vi "Untitled 1.vi"   [LabVIEW 2014]
uses:
  <vilib>/FTP/NI_FTP.lvlib
types:
  T1 = typedef "NI_FTP.lvlib/FTP Session.ctl" = refnum<k5>
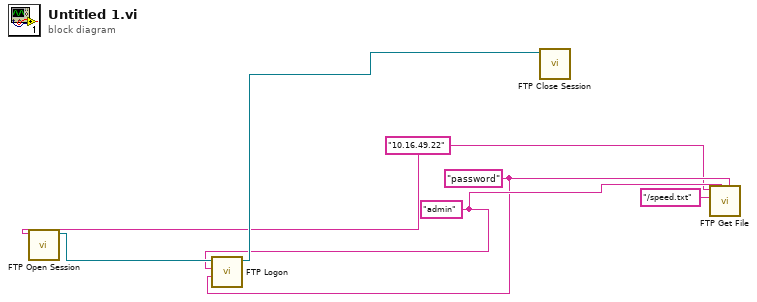
[diagram p0: block diagram]
diagram:
  w2 = "10.16.49.22" ("host")
  w3 = "password" ("password")
  w4 = "admin" ("user")
  n1 = call <vilib>:"FTP Open Session.vi"("address"=w2) -> ("ftp session"=w6:T1)  [unwired: 7 in, 3 out]
  n2 = call <vilib>:"FTP Logon.vi"("password"=w3, "user"=w4, "ftp session"=w6) -> ("ftp session out"=w5:T1)  [unwired: 5 in, 3 out]
  n3 = call <vilib>:"FTP Close Session.vi"("ftp session"=w5) -> ()  [unwired: 7 in, 4 out]
  n4 = call <vilib>:"FTP Get File.vi"("password"=w3, "user"=w4, "remote path"="/speed.txt", "host"=w2) -> ()  [unwired: 6 in, 2 out]
